vi "AlliGator Load Experimental IRF.vi"(8 "error in":errorcluster, 9 "Experimental IRF Loaded?":bool, 10 "Plot Data in":T1, 11 "XYGraph in":refnum<vi>) -> (0 "error out":errorcluster, 1 "Experimental IRF Loaded?":bool, 2 "Plot Data out":T1, 4 "Message":string)   [LabVIEW 2021, in "AlliGator Fit Method Benchmark.lvlib"]
doc: "Load experimental IRF from ASCII file."
uses:
  AlliGator Fit Method Benchmark.lvlib
  Graphs/XY Graph/XY Plot Data.ctl
  Graphs/XY Graph/XY Graph Add-Ons.lvlib
panel:
  # "see the AlliGator License on the block diagram (Ctrl+E or Window:Show Block Diagram)"
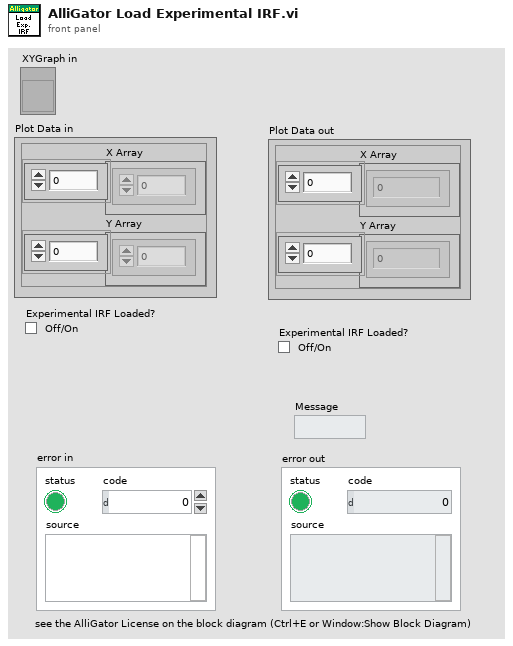
[diagram p1: front panel]
types:
  T1 = typedef "XY Graph Add-Ons.lvlib/XY Plot Data.ctl" = cluster{"X Array":dbl[], "Y Array":dbl[]}
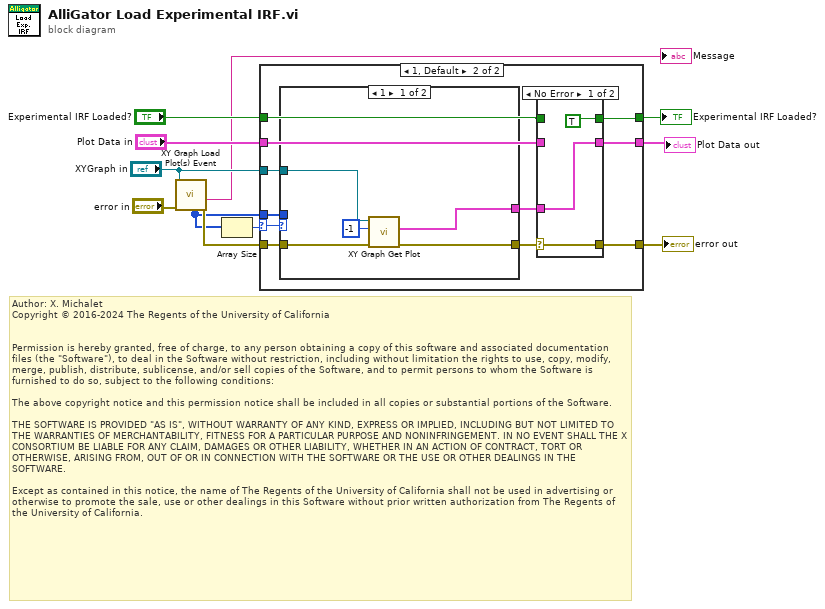
[diagram p0: block diagram]
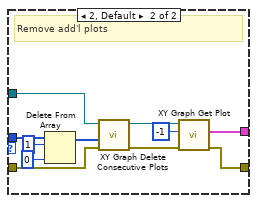
[diagram p4: hidden frame]
diagram:
  # "Author: X. Michalet\nCopyright © 2016-2024 The Regents of the University of California\n \n\nPermission is hereby granted, free of charge, to any person obtaining a copy of this software and associated documentation files (the \"Software\"), to deal in the Software without restriction, including without limitation the rights to use, copy, modify, merge, publish, distribute, sublicense, and/or sell copies of the Software, and to permit persons to whom the Software is furnished to do so, subject to the following conditions:\n\nThe above copyright notice and this permission notice shall be included in all copies or substantial portions of the Software.\n\nTHE SOFTWARE IS PROVIDED \"AS IS\", WITHOUT WARRANTY OF ANY KIND, EXPRESS OR IMPLIED, INCLUDING BUT NOT LIMITED TO THE WARRANTIES OF MERCHANTABILITY, FITNESS FOR A PARTICULAR PURPOSE AND NONINFRINGEMENT. IN NO EVENT SHALL THE X CONSORTIUM BE LIABLE FOR ANY CLAIM, DAMAGES OR OTHER LIABILITY, WHETHER IN AN ACTION OF CONTRACT, TORT OR OTHERWISE, ARISING FROM, OUT OF OR IN CONNECTION WITH THE SOFTWARE OR THE USE OR OTHER DEALINGS IN THE SOFTWARE.\n\nExcept as contained in this notice, the name of The Regents of the University of California shall not be used in advertising or otherwise to promote the sale, use or other dealings in this Software without prior written authorization from The Regents of the University of California."
  n1 = call "XY Graph Load Plot(s) Event.vi"("Error In"="error in", "XYGraph Ref"="XYGraph in") -> ("Error Out"=w6:errorcluster, "Message"=→"Message":string, "# Plots Added"=w4:i32[])  [unwired: 4 in, 3 out]
  n2 = Array Size(array=w4) -> (size(s)=w3:i32)
  n3 = case shown="1, Default" w3 {
    selector: w3 -> [_ w22]
    tunnel: w4 -> [_ w25]
    tunnel: "XYGraph in" -> [_ w24]
    tunnel: w6 -> [w14 w23]
    tunnel: [w14 w20] -> w7
    tunnel: "Plot Data in" -> [w13 w16]
    tunnel: [w13 w19] -> w9
    tunnel: "Experimental IRF Loaded?" -> [w12 w17]
    tunnel: [w12 w18] -> w11
    frame 0 {
    }
    frame 1, Default {
      n4 = case shown="1" w22 {
        tunnel: w25 -> [_ w47]
        tunnel: w24 -> [w35 w43]
        tunnel: w23 -> [w36 w42]
        tunnel: [w34 w39] -> w15
        tunnel: [w33 w38] -> w21
        frame 1 {
          n5 = call "XY Graph Get Plot.vi"("error in (no error)"=w36, "Plot Index (-1: last)"=-1, "XYGraph in"=w35) -> ("error out"=w33:errorcluster, "Plot Data"=w34:T1)  [unwired: 4 in, 3 out]
        }
        frame 2, Default {
          # "Remove add'l plots"
          n6 = Delete From Array(array=w47, length=1, index=0) -> (array with subset deleted=w44:i32[])  [unwired: 1 out]
          n7 = call "XY Graph Delete Consecutive Plots.vi"("Error In"=w42, "Plot Indices"=w44, "XYGraph Ref"=w43) -> ("Error Out"=w41:errorcluster, "XYGraph Ref"=w40:refnum<vi>)  [unwired: 5 in, 2 out]
          n8 = call "XY Graph Get Plot.vi"("error in (no error)"=w41, "Plot Index (-1: last)"=-1, "XYGraph in"=w40) -> ("error out"=w38:errorcluster, "Plot Data"=w39:T1)  [unwired: 4 in, 3 out]
        }
      }
      n9 = case shown="No Error" w21 {
        selector: w21 -> [w28 w30]
        tunnel: [w26 w29] -> w19
        tunnel: w17 -> [_ w31]
        tunnel: [TRUE w31] -> w18
        tunnel: [w28 w30] -> w20
        tunnel: w16 -> [_ w29]
        tunnel: w15 -> [w26 _]
        frame No Error {
        }
        frame Error {
        }
      }
    }
  }
  "Experimental IRF Loaded?" <- w11
  "Plot Data out" <- w9
  "error out" <- w7
